vi "HeaderAction.vi"(0 "SR830In":refnum<class "SR830.lvclass"> caption="DNL_LabVIEW Object in", 11 "ErrIn (NoErr)":errorcluster caption="entrée d'erreur (pas d'erreur)") -> (4 "SR830Out":refnum<class "SR830.lvclass"> caption="DNL_LabVIEW Object out", 6 "DataNames":string[](array[string]), 8 "Instr Name":string, 10 "HeaderString":string, 14 "DisplayNames":string[](array[string]), 15 "error out":errorcluster caption="sortie d'erreur")   [LabVIEW 2012, in "SR830.lvclass"]
uses:
  SR830.lvclass
  SR830.lvclass/SR830.ctl
  BaseDevice/BaseDevice.lvclass
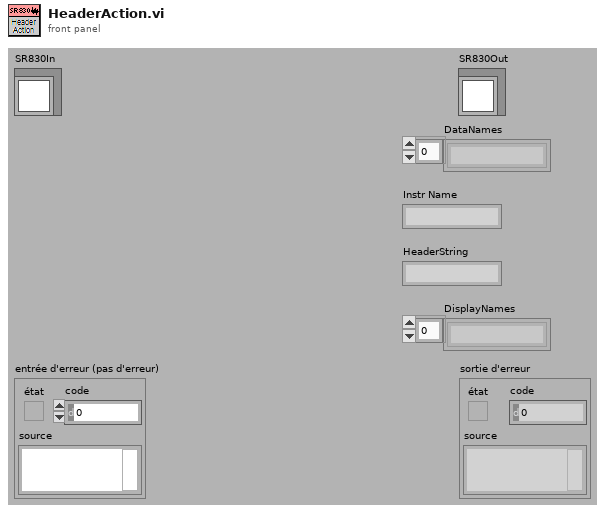
[diagram p1: front panel]
types:
  T1 = enum16{"Phase Shift", "Reference Source", "Reference Frequency", "Reference Trigger", "Detection Harmonic", "Sine Amplitude", "Input Configuration", "Input Shield", "Input Coupling", "Input Line Notch Filter", "Sensitivity", "Dynamic Reserve", "Time Constant", "Low Pass Filter", "Sync Filter", "Expand X", "Expand Y", "Expand R", "All"}
  T2 = typedef "SR830.lvclass/SR830_Func.ctl" = enum16{"Read X & Y (V,V)", "Read Mag & Phase (V,°)", "Read X,Y,Mag & Phase (V,V,V,°)", "Read THz Pump Off/On (V,V,V,°,V,V,V,°,V)"}
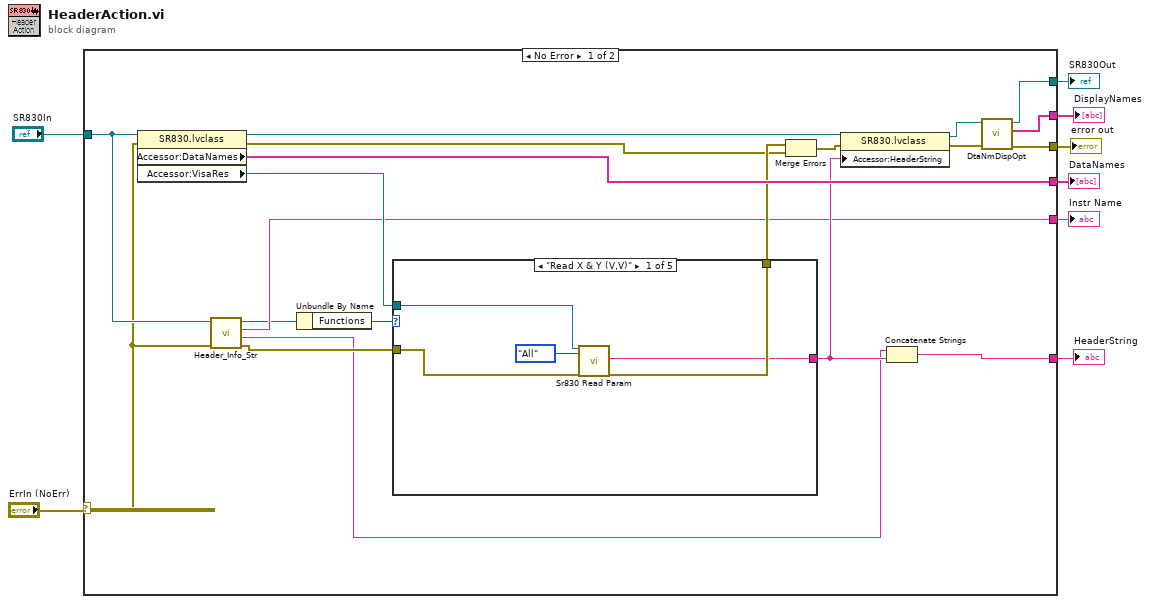
[diagram p0: block diagram]
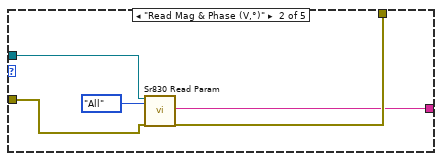
[diagram p2: hidden frame]
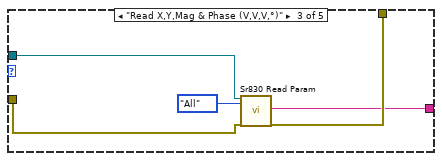
[diagram p3: hidden frame]
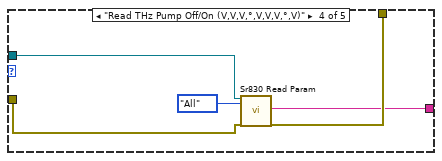
[diagram p4: hidden frame]
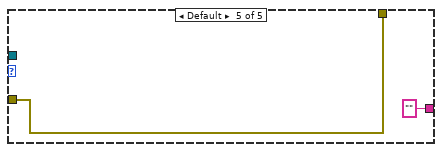
[diagram p5: hidden frame]
diagram:
  n1 = case shown="No Error" "ErrIn (NoErr)" {
    selector: "ErrIn (NoErr)" -> [w14 w51]
    tunnel: [w10 _] -> w7
    tunnel: [w28 _] -> w6
    tunnel: "SR830In" -> [w17 w52]
    tunnel: [w22 w51] -> w4
    tunnel: [w18 w52] -> w3
    tunnel: [w16 _] -> w2
    tunnel: [w19 _] -> w1
    frame No Error {
      n2 = property class="SR830.lvclass"(reference=w17, error in=w14) -> (reference out=w27:refnum<class "SR830.lvclass">, error out=w11:errorcluster, "Accessor:DataNames"=w28:string[], "Accessor:VisaRes"=w25:refnum<visa-resource-name>)
      n3 = call "Header_Info_Str.vi"("error in (no error)"=w14, "Sr830 in"=w17) -> ("error out"=w13:errorcluster, "HdrInfoStr"=w9:string, "InstrumentName"=w16:string, "Sr830 out"=w15:refnum<class "SR830.lvclass">)  [unwired: 6 in]
      n4 = Unbundle By Name(w15) -> ("Functions"=w26:T2)
      n5 = case shown="\"Read X & Y (V,V)\"" w26 {
        tunnel: w25 -> [w33 w38 w43 w48 _]
        tunnel: w13 -> [w29 w34 w41 w46 w49]
        tunnel: [w31 w36 w40 w45 w49] -> w24
        tunnel: [w30 w35 w39 w44 "" ("Params")] -> w23
        frame "Read X & Y (V,V)" {
          n6 = call <userlib>:"Sr830 Read Param.vi"("Ressource VISA"=w33, "Énum"=T1."All", "error in (no error)"=w29) -> ("Params"=w30:string, "error out"=w31:errorcluster)  [unwired: 13 in, 2 out]
        }
        frame "Read Mag & Phase (V,°)" {
          n7 = call <userlib>:"Sr830 Read Param.vi"("Ressource VISA"=w38, "Énum"=T1."All", "error in (no error)"=w34) -> ("Params"=w35:string, "error out"=w36:errorcluster)  [unwired: 13 in, 2 out]
        }
        frame "Read X,Y,Mag & Phase (V,V,V,°)" {
          n8 = call <userlib>:"Sr830 Read Param.vi"("Ressource VISA"=w43, "Énum"=T1."All", "error in (no error)"=w41) -> ("Params"=w39:string, "error out"=w40:errorcluster)  [unwired: 13 in, 2 out]
        }
        frame "Read THz Pump Off/On (V,V,V,°,V,V,V,°,V)" {
          n9 = call <userlib>:"Sr830 Read Param.vi"("Ressource VISA"=w48, "Énum"=T1."All", "error in (no error)"=w46) -> ("Params"=w44:string, "error out"=w45:errorcluster)  [unwired: 13 in, 2 out]
        }
        frame Default {
        }
      }
      n10 = Merge Errors(w24, w11) -> (w12:errorcluster)
      n11 = property class="SR830.lvclass"(reference=w27, error in=w12, "Accessor:HeaderString"=w23) -> (reference out=w20:refnum<class "SR830.lvclass">, error out=w21:errorcluster)
      n12 = Concatenate Strings(w9, w23) -> (w10:string)
      n13 = call "DtaNmDispOpt.vi"("error in (no error)"=w21, "BaseDevice en entrée"=w20) -> ("error out"=w22:errorcluster, "DisplayNames"=w19:string[], "BaseDevice en sortie"=w18:refnum<class "SR830.lvclass">)  [unwired: 7 in]
    }
    frame Error {
    }
  }
  "error out" <- w4
  "SR830Out" <- w3
  "DataNames" <- w6
  "HeaderString" <- w7
  "Instr Name" <- w2
  "DisplayNames" <- w1
